vi "Problem2.4.vi"() -> ()   [LabVIEW 2019]
panel:
  out "Timer Done":bool
  in  "Wait Time (Seconds)":dbl=4.0
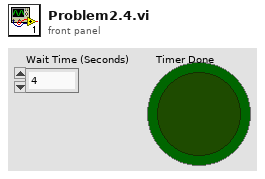
[diagram p1: front panel]
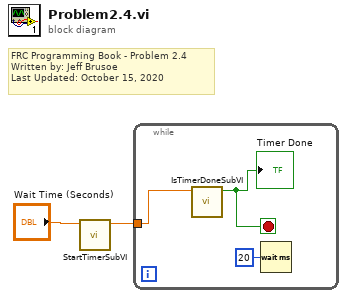
[diagram p0: block diagram]
diagram:
  # "FRC Programming Book - Problem 2.4\nWritten by: Jeff Brusoe\nLast Updated: October 15, 2020"
  n1 = call "StartTimerSubVI.vi"("Wait Time (Seconds)"="Wait Time (Seconds)") -> ("End Time (Seconds)"=w2:dbl)  [unwired: 10 in]
  n2 = while {
    tunnel: w2 -> [w4]
    stop <- w3 stop-if-true
    n3 = call "IsTimerDoneSubVI.vi"("End Time (Seconds)"=w4) -> ("Time Done"=w3:bool)  [unwired: 8 in]
    "Timer Done" <- w3
    n4 = Wait (ms)(milliseconds to wait=u32 20) -> ()  [unwired: 1 out]
  }
